vi "sub_Check Error Folder.vi"(8 "error in (no error)":errorcluster) -> (0 "error out":errorcluster)   [LabVIEW 2016, in "System.lvlib"]
uses:
  System.lvlib
  <vilib>/Utility/sysdir.llb/System Directory Type.ctl
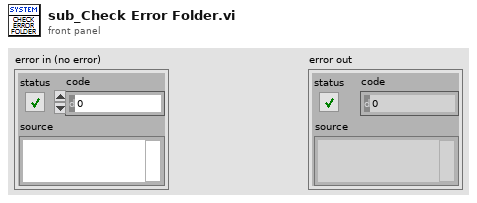
[diagram p1: front panel]
types:
  T1 = typedef "System Directory Type.ctl" = i32
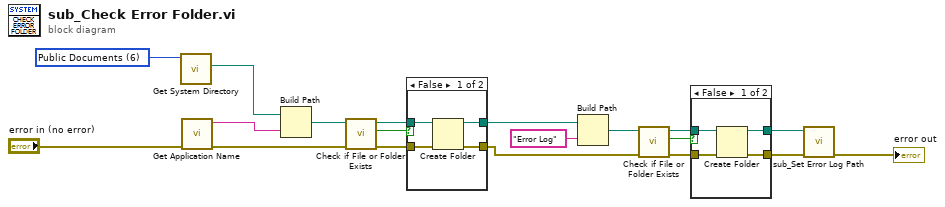
[diagram p0: block diagram]
diagram:
  w19 = T1 6 items=["User Home"=0, "User Desktop"=1, "User Documents"=2, "User Application Data"=3, "User Preferences"=4, "User Temporary"=5, "Public Documents"=6, "Public Application Data"=7, "Public Preferences"=8, "Public Cache"=13, "System Core Libraries"=9, "System Installed Libraries"=10, "Application Files"=11, "Boot Volume Root"=12] ("system directory type")
  n1 = call <vilib>:"Get System Directory.vi"("system directory type"=w19) -> ("system directory"=w18:path)  [unwired: 10 in]
  n2 = call "Get Application Name.vi"("error in (no error)"="error in (no error)") -> ("error out"=w5:errorcluster, "Application Name"=w4:string)  [unwired: 9 in]
  n3 = Build Path(base path=w18, name or relative path=w4) -> (appended path=w17:path)
  n4 = call <vilib>:"Check if File or Folder Exists.vi"("error in (no error)"=w5, "path"=w17) -> ("error out"=w9:errorcluster, "file or folder exists?"=w16:bool, "dup path"=w15:path)  [unwired: 7 in]
  n5 = case shown="False" w16 {
    tunnel: w15 -> [w22 w25]
    tunnel: [w23 w25] -> w14
    tunnel: w9 -> [w21 w24]
    tunnel: [w20 w24] -> w8
    frame False {
      n6 = Create Folder(path (use dialog)=w22, error in=w21) -> (created path=w23:path, error out=w20:errorcluster)  [unwired: 1 in, 1 out]
    }
    frame True {
    }
  }
  n7 = Build Path(base path=w14, name or relative path="Error Log") -> (appended path=w10:path)
  n8 = call <vilib>:"Check if File or Folder Exists.vi"("error in (no error)"=w8, "path"=w10) -> ("error out"=w7:errorcluster, "file or folder exists?"=w11:bool, "dup path"=w12:path)  [unwired: 7 in]
  n9 = case shown="False" w11 {
    tunnel: w12 -> [w28 w31]
    tunnel: [w29 w31] -> w3
    tunnel: w7 -> [w27 w30]
    tunnel: [w26 w30] -> w2
    frame False {
      n10 = Create Folder(path (use dialog)=w28, error in=w27) -> (created path=w29:path, error out=w26:errorcluster)  [unwired: 1 in, 1 out]
    }
    frame True {
    }
  }
  n11 = call "sub_Set Error Log Path.vi"("error in (no error)"=w2, "Path"=w3) -> ("error out"=→"error out":errorcluster)  [unwired: 9 in]
